vi "Get Statistics.vi"(8 "error in (no error)":errorcluster, 11 "Result Model in":refnum<class "Result Model by Reference.lvclass">) -> (0 "error out":errorcluster, 2 "Results":T1)   [LabVIEW 2020, in "Result Model by Reference.lvclass"]
uses:
  Result Model by Reference.lvclass
  Result Model/Statistics.ctl
  Result Model by Reference.lvclass/Result Model by Reference.ctl
  Result Model/Result Model.lvclass
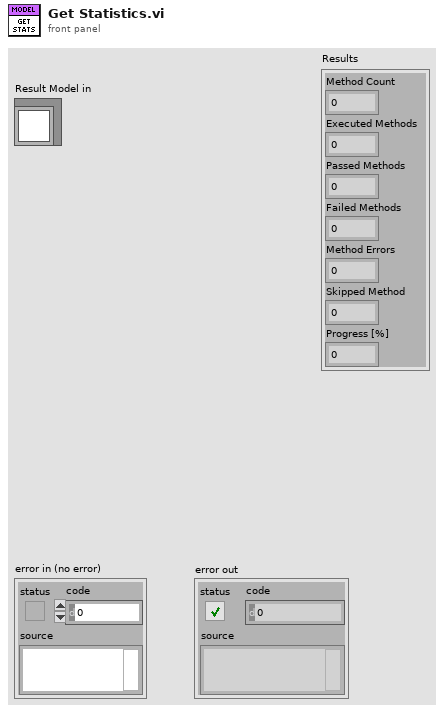
[diagram p1: front panel]
types:
  T1 = typedef "Result Model.lvclass/Statistics.ctl" = cluster{"Method Count":u32, "Executed Methods":u32, "Passed Methods":u32, "Failed Methods":u32, "Method Errors":u32, "Skipped Method":u32, "Progress [%]":dbl}
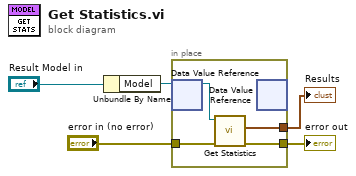
[diagram p0: block diagram]
diagram:
  n1 = Unbundle By Name("Result Model in") -> ("Model"=w5:refnum<data-value>)
  n2 = in-place {
    in-place-border: [w9] -> w3
    in-place-border: "error in (no error)" -> [w7]
    in-place-border: [w6] -> w1
    n3 = in-place-dvr #1(w5) -> (w8:refnum<class "Result Model.lvclass">)  [unwired: 1 out]
    n4 = call "Get Statistics.vi"("error in (no error)"=w7, "Result Model in"=w8) -> ("error out"=w9:errorcluster, "Results"=w6:T1)  [unwired: 8 in]
    n5 = in-place-dvr #1() -> ()  [unwired: 1 in, 2 out]
  }
  "error out" <- w3
  "Results" <- w1
